vi "DrawChessboardRadon.vi"(6 "Marker Locations":T4[](array[typedef]), 8 "error in (no error)":errorcluster, 10 "Chessboard Corners Info":T3, 11 "Target Size":T2) -> (0 "error out":errorcluster, 3 "image data":T1)   [LabVIEW 2020, in "g_ar_toolkit.feature_detection.lvlib"]
uses:
  g_ar_toolkit.feature_detection.lvlib
  Chessboard Square Marker.ctl
  Chessboard Corner Info.ctl
  g_ar_toolkit.common/Image Size (Integer).ctl
  <vilib>/picture/picture.llb/imagedata.ctl
  ChessboardSquareLocation.ctl
  g_ar_toolkit.common/g_ar_toolkit.common.lvlib
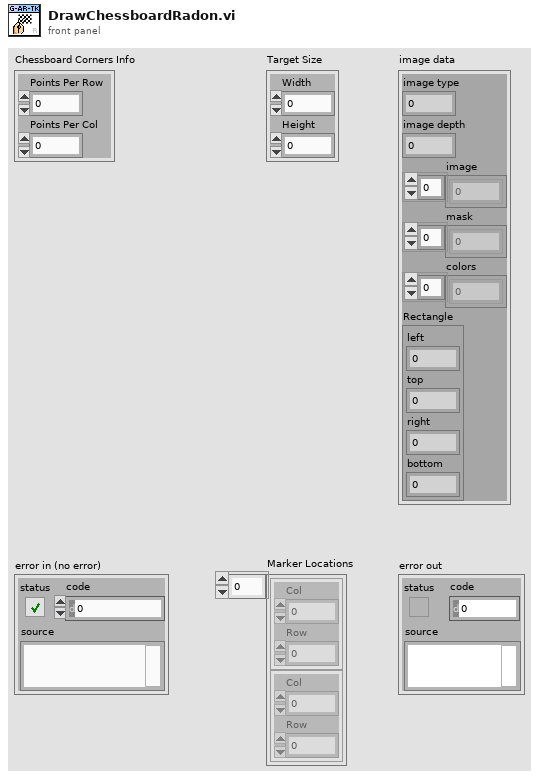
[diagram p1: front panel]
types:
  T1 = typedef "imagedata.ctl" = cluster{"image type":i32, "image depth":i32, "image":u8[], "mask":u8[], "colors":u32[], "Rectangle":cluster{"left":i16, "top":i16, "right":i16, "bottom":i16}}
  T2 = typedef "g_ar_toolkit.common.lvlib/Image Size (Integer).ctl" = cluster{"Width":u16, "Height":u16}
  T3 = typedef "g_ar_toolkit.feature_detection.lvlib/Chessboard Corner Info.ctl" = cluster{"Points Per Row":u8, "Points Per Col":u8}
  T4 = typedef "g_ar_toolkit.feature_detection.lvlib/Chessboard Square Marker.ctl" = cluster{"Col":u8, "Row":u8}
  T5 = typedef "g_ar_toolkit.feature_detection.lvlib/ChessboardSquareLocation.ctl" = enum16{"Top Left Corner", "Top Row", "Top Right Corner ", "Left Col", "Right Col", "Bottom Left Corner", "Bottom Row", "Bottom Right Corner", "Other"}
  T6 = map{cluster{"First Row":bool, "Last Row":bool, "First Col":bool, "Last Col":bool}, T5}
  T7 = cluster{"Position":cluster{"First Row":bool, "Last Row":bool, "First Col":bool, "Last Col":bool}, "f":T5}[]
  T8 = cluster{"First Row":bool, "Last Row":bool, "First Col":bool, "Last Col":bool}
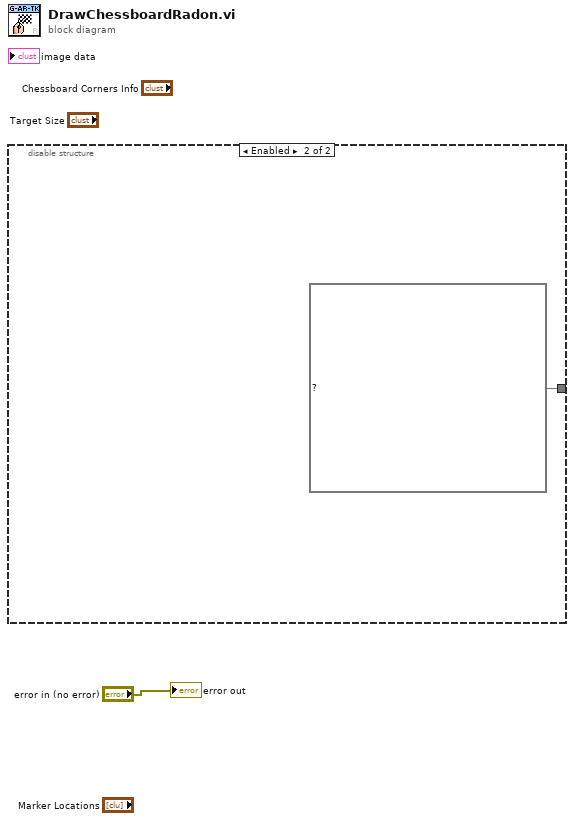
[diagram p0: block diagram]
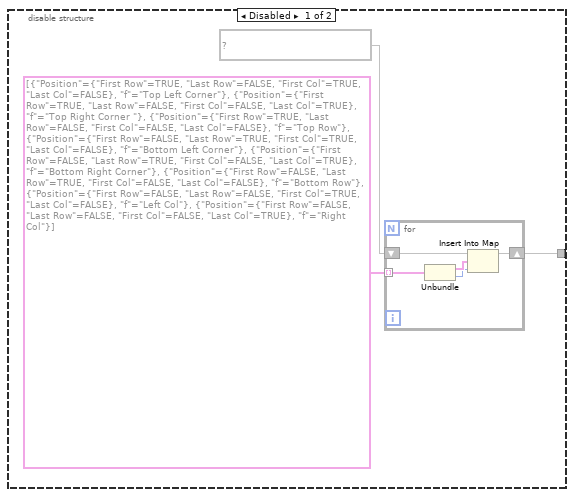
[diagram p2: hidden frame]
diagram:
  n1 = disable-structure shown="Enabled" {
    disable-tunnel: [w2 T6 {{"First Row"=FALSE, "Last Row"=FALSE, "First Col"=FALSE, "Last Col"=TRUE}=enum."Right Col", {"First Row"=FALSE, "Last Row"=FALSE, "First Col"=TRUE, "Last Col"=FALSE}=enum."Left Col", {"First Row"=FALSE, "Last Row"=TRUE, "First Col"=FALSE, "Last Col"=FALSE}=enum."Bottom Row", {"First Row"=FALSE, "Last Row"=TRUE, "First Col"=FALSE, "Last Col"=TRUE}=enum."Bottom Right Corner", {"First Row"=FALSE, "Last Row"=TRUE, "First Col"=TRUE, "Last Col"=FALSE}=enum."Bottom Left Corner", {"First Row"=TRUE, "Last Row"=FALSE, "First Col"=FALSE, "Last Col"=FALSE}=enum."Top Row", {"First Row"=TRUE, "Last Row"=FALSE, "First Col"=FALSE, "Last Col"=TRUE}=enum."Top Right Corner ", {"First Row"=TRUE, "Last Row"=FALSE, "First Col"=TRUE, "Last Col"=FALSE}=enum."Top Left Corner"} ("Map")] -> _
    frame Disabled {
      n2 = for {
        tunnel: T7 [{"Position"={"First Row"=TRUE, "Last Row"=FALSE, "First Col"=TRUE, "Last Col"=FALSE}, "f"=enum."Top Left Corner"}, {"Position"={"First Row"=TRUE, "Last Row"=FALSE, "First Col"=FALSE, "Last Col"=TRUE}, "f"=enum."Top Right Corner "}, {"Position"={"First Row"=TRUE, "Last Row"=FALSE, "First Col"=FALSE, "Last Col"=FALSE}, "f"=enum."Top Row"}, {"Position"={"First Row"=FALSE, "Last Row"=TRUE, "First Col"=TRUE, "Last Col"=FALSE}, "f"=enum."Bottom Left Corner"}, {"Position"={"First Row"=FALSE, "Last Row"=TRUE, "First Col"=FALSE, "Last Col"=TRUE}, "f"=enum."Bottom Right Corner"}, {"Position"={"First Row"=FALSE, "Last Row"=TRUE, "First Col"=FALSE, "Last Col"=FALSE}, "f"=enum."Bottom Row"}, {"Position"={"First Row"=FALSE, "Last Row"=FALSE, "First Col"=TRUE, "Last Col"=FALSE}, "f"=enum."Left Col"}, {"Position"={"First Row"=FALSE, "Last Row"=FALSE, "First Col"=FALSE, "Last Col"=TRUE}, "f"=enum."Right Col"}] -> [w9] mode=indexing
        shift-right: [w6] -> w2
        shift-left: T6 {} ("Size: 0") -> [w5]
        n3 = Unbundle(w9) -> ("Position"=w8:T8, "f"=w7:T5)
        n4 = Insert Into Map(map in=w5, key=w8, value=w7) -> (map out=w6:T6)  [unwired: 2 out]
      }
    }
    frame Enabled {
    }
  }
  "error out" <- "error in (no error)"
